vi "Control Panel.vi"(8 "error in (no error)":errorcluster, 11 "Fake Fluke Multimeter in":refnum<class "Fluke Multimeter.lvclass">) -> (0 "error out":errorcluster, 3 "Fake Fluke Multimeter out":refnum<class "Fluke Multimeter.lvclass">)   [LabVIEW 2017, in "Fluke Multimeter.lvclass"]
doc: "(Dynamic) A user-level application that simulates the physical front panel of the Instrument. Provide the user with buttons to manually control features of the instrument, and provide indicators of its current state."
uses:
  Fluke Multimeter.lvclass
  Fluke Multimeter.lvclass/Fluke Multimeter.ctl
  Fluke 8840/Fluke 8840.lvlib
  Utility Classes/Readable/Readable.lvclass
panel:
  out "AutoRange":bool
  out "unit":string
  in  "Reset":bool
  in  "Read Current Value":bool
  out "Value":dbl
  in  "Set":bool
  in  "Read to Control":bool
  in  "Read":bool
  in  "trigger mode set":u16(ring) items=["internal - continuous trigger", "external - rear panel trigger with delay", "external - bus trigger with delay", "external - rear panel trigger", "external - bus trigger"]
  in  "rate set":u16(ring) items=["slow", "medium", "fast"]
  in  "range set":u16(ring)=6 items=["autorange", "200mV, 200 ohms", "2V, 2 kohms", "20V, 20 kohms", "200V, 200 kohms", "1000Vdc, 700 Vac, 2 Mohms", "20 Mohms"]
  in  "function set":u16(ring) items=["volts DC", "volts AC", "2-wire k.ohms", "4-wire k.ohms", "mA DC", "mA AC"]
  out "trigger mode":u16(ring) items=["internal - continuous trigger", "external - rear panel trigger with delay", "external - bus trigger with delay", "external - rear panel trigger", "external - bus trigger"]
  out "rate":u16(ring) items=["slow", "medium", "fast"]
  out "range":u16(ring)=6 items=["autorange", "200mV, 200 ohms", "2V, 2 kohms", "20V, 20 kohms", "200V, 200 kohms", "1000Vdc, 700 Vac, 2 Mohms", "20 Mohms"]
  out "function":u16(ring) items=["volts DC", "volts AC", "2-wire k.ohms", "4-wire k.ohms", "mA DC", "mA AC"]
  in  "stop":bool
  in  "Copy actual to set":bool
  in  "Populate fields with member data":bool
  # "Note: can't set trigger mode yet. Apparently need to create driver for the Y1 command"
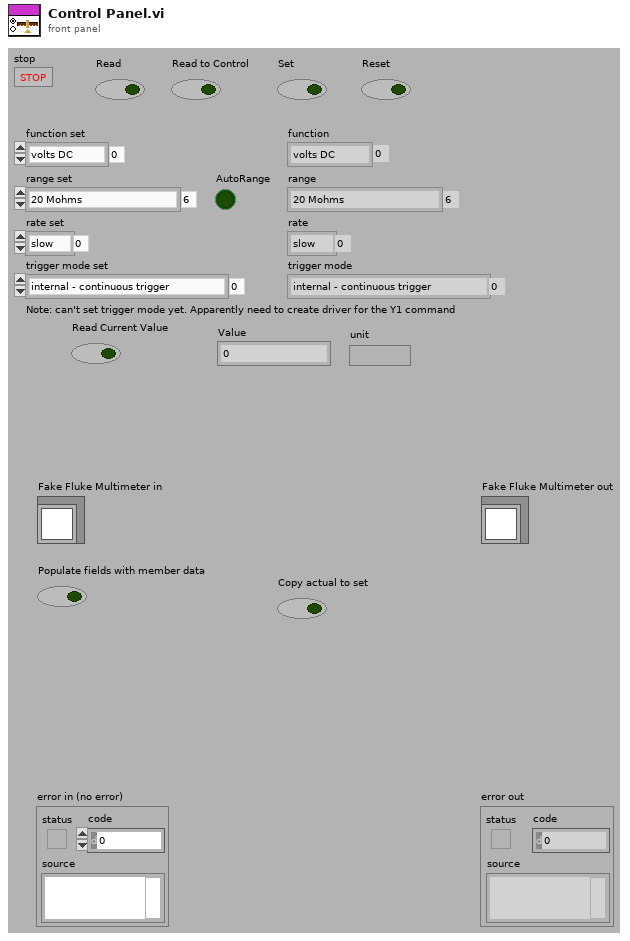
[diagram p1: front panel]
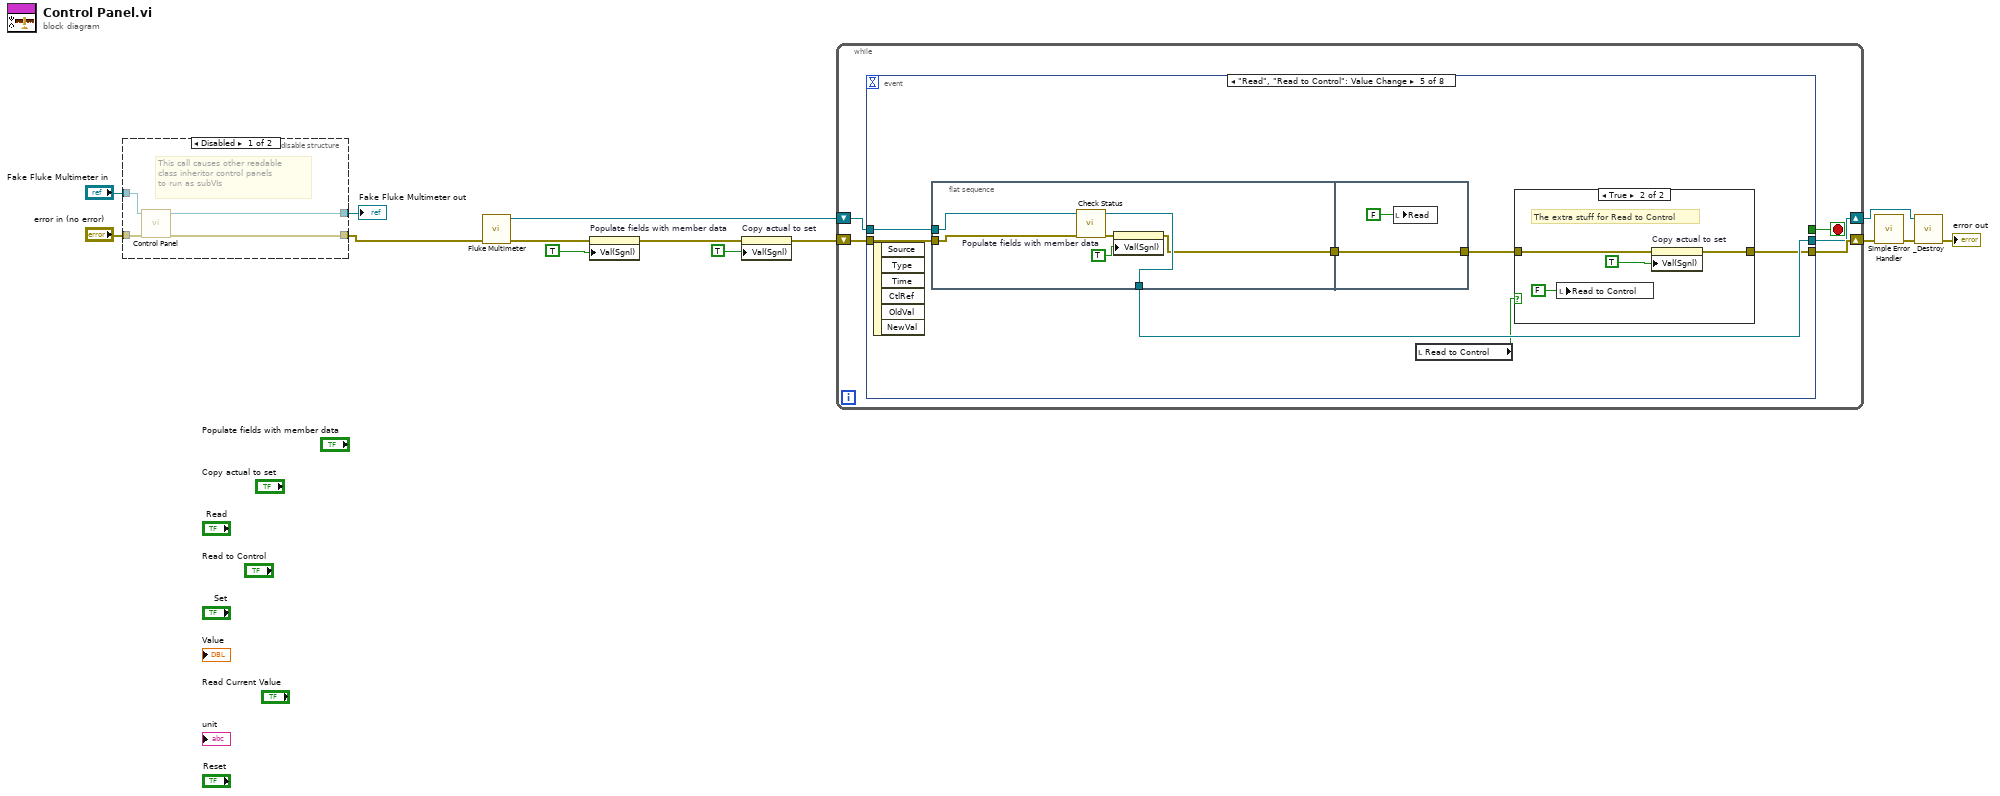
[diagram p0: block diagram]
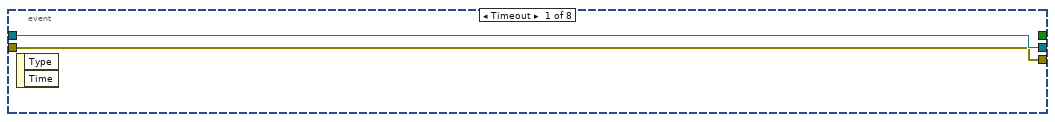
[diagram p3: hidden frame]
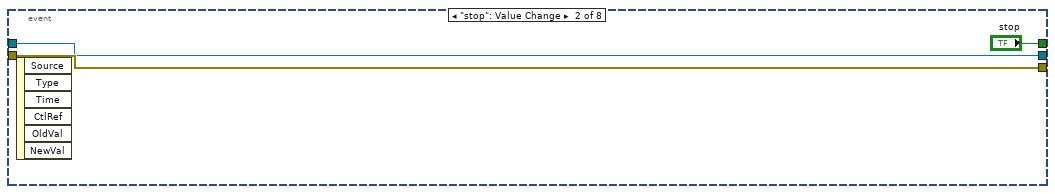
[diagram p4: hidden frame]
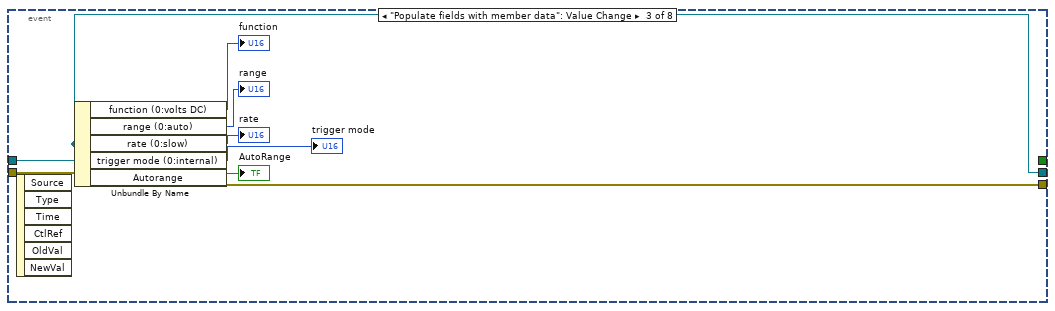
[diagram p5: hidden frame]
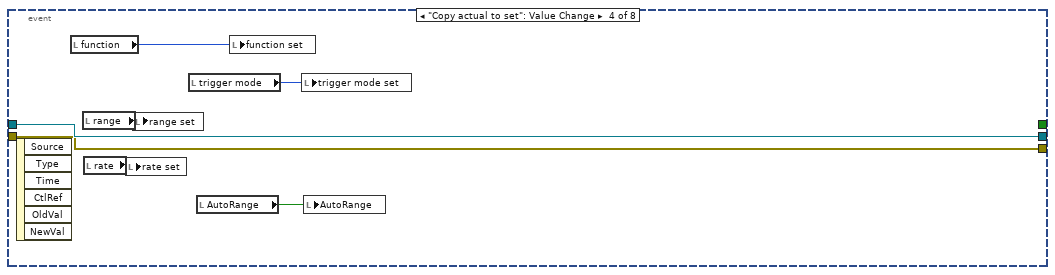
[diagram p6: hidden frame]
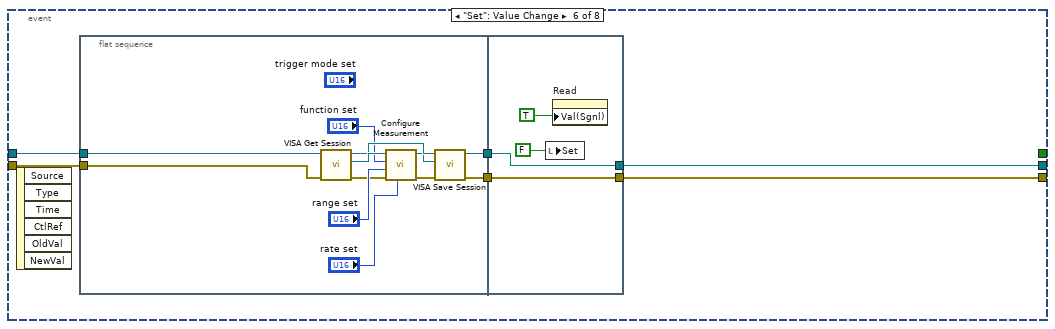
[diagram p8: hidden frame]
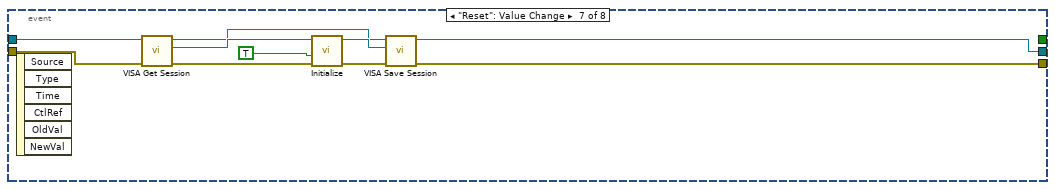
[diagram p9: hidden frame]
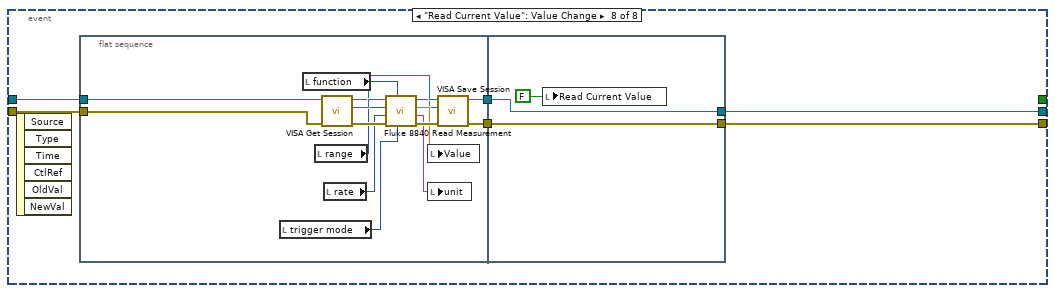
[diagram p10: hidden frame]
diagram:
  n1 = disable-structure shown="Disabled" {
    disable-tunnel: [w18 w20] -> w14
    disable-tunnel: "error in (no error)" -> [w17 w19]
    disable-tunnel: "Fake Fluke Multimeter in" -> [w16 w20]
    disable-tunnel: [w15 w19] -> w11
    frame Disabled {
      # "This call causes other readable\nclass inheritor control panels\nto run as subVIs"
      n2 = call-parent "Control Panel.vi"("error in (no error)"=w17, "Instrument in"=w16) -> ("error out"=w15:errorcluster, "Instrument out"=w18:refnum<class "Fluke Multimeter.lvclass">)  [unwired: 8 out]
    }
    frame Enabled {
    }
  }
  "Fake Fluke Multimeter out" <- w14
  n3 = call "Fluke Multimeter.vi"("error in (no error)"=w11) -> ("error out"=w10:errorcluster, "Fluke Multimeter out"=w7:refnum<class "Fluke Multimeter.lvclass">)  [unwired: 9 out]
  n4 = property on="Populate fields with member data" class="Bool (strict)"(error in=w10, "Val(Sgnl)"=TRUE ("Value (Signaling)")) -> (error out=w9:errorcluster)  [unwired: 1 in, 1 out]
  n5 = property on="Copy actual to set" class="Bool (strict)"(error in=w9, "Val(Sgnl)"=TRUE ("Value (Signaling)")) -> (error out=w8:errorcluster)  [unwired: 1 in, 1 out]
  n6 = while {
    shift-right: [w22] -> w5
    shift-left: w7 -> [w21]
    shift-right: [w24] -> w2
    shift-left: w8 -> [w23]
    stop <- w25 stop-if-true
    n7 = event shown="[4] \"Read\", \"Read to Control\": Value Change" {
      selector: _ -> [_ _ _ _ _ _ _ _]
      dyn-events: _ -> [_ _ _ _ _ _ _ _]
      timeout: _ -> [_ _ _ _ _ _ _ _]
      tunnel: [_ "stop" _ _ _ _ _ _] -> w25
      tunnel: [w26 w29 w32 w39 w45 w67 w88 w100] -> w24
      tunnel: w23 -> [w26 w29 w32 w39 w51 w69 w93 w99]
      tunnel: [w27 w28 w33 w40 w49 w68 w87 w101] -> w22
      tunnel: w21 -> [w27 w28 w33 w40 w50 w70 w94 w102]
      event Timeout {
        n8 = event-data() -> ()  [unwired: 3 out]
      }
      event "stop": Value Change {
        n9 = event-data() -> ()  [unwired: 7 out]
      }
      event "Populate fields with member data": Value Change {
        n10 = event-data() -> ()  [unwired: 7 out]
        n11 = Unbundle By Name(w33) -> ("function (0:volts DC)"=→"function":u16, "range (0:auto)"=→"range":u16, "rate (0:slow)"=→"rate":u16, "trigger mode (0:internal)"=→"trigger mode":u16, "Autorange"=→"AutoRange":bool)
      }
      event "Copy actual to set": Value Change {
        n12 = event-data() -> ()  [unwired: 7 out]
        n13 = local read "function"() -> (w44:u16)
        n14 = local read "range"() -> (w43:u16)
        n15 = local read "rate"() -> (w42:u16)
        n16 = local write "rate set"(w42) -> ()
        n17 = local write "range set"(w43) -> ()
        n18 = local read "trigger mode"() -> (w41:u16)
        n19 = local read "AutoRange"() -> (w38:bool)
        n20 = local write "function set"(w44) -> ()
        n21 = local write "trigger mode set"(w41) -> ()
        n22 = local write "AutoRange"(w38) -> ()
      }
      event "Read", "Read to Control": Value Change {
        n23 = event-data() -> ()  [unwired: 7 out]
        n24 = flat-sequence {
          tunnel: w51 -> [w62]
          tunnel: w50 -> [w61]
          tunnel: [w60] -> w49
          tunnel: [w57] -> w46
          tunnel: [w63] -> w47
          tunnel: w46 -> [w63]
          frame #0 {
            n25 = call-dynamic "Check Status.vi"("error in (no error)"=w62, "Fluke Multimeter in"=w61) -> ("error out"=w59:errorcluster, "Fluke Multimeter out"=w60:refnum<class "Fluke Multimeter.lvclass">)  [unwired: 8 out]
            n26 = property on="Populate fields with member data" class="Bool (strict)"(error in=w59, "Val(Sgnl)"=TRUE ("Value (Signaling)")) -> (error out=w57:errorcluster)  [unwired: 1 in, 1 out]
          }
          frame #1 {
            n27 = local write "Read"(FALSE ("Read")) -> ()
          }
        }
        n28 = local read "Read to Control"() -> (w48:bool)
        n29 = case shown="True" w48 {
          tunnel: w47 -> [w52 w54]
          tunnel: [w52 w53] -> w45
          frame False {
          }
          frame True {
            # "The extra stuff for Read to Control"
            n30 = local write "Read to Control"(FALSE ("Read to Control")) -> ()
            n31 = property on="Copy actual to set" class="Bool (strict)"(error in=w54, "Val(Sgnl)"=TRUE ("Value (Signaling)")) -> (error out=w53:errorcluster)  [unwired: 1 in, 1 out]
          }
        }
      }
      event "Set": Value Change {
        n32 = event-data() -> ()  [unwired: 7 out]
        n33 = flat-sequence {
          tunnel: w70 -> [w82]
          tunnel: w69 -> [w81]
          tunnel: [w78] -> w66
          tunnel: [w71] -> w65
          tunnel: [w85] -> w67
          tunnel: [w86] -> w68
          tunnel: w66 -> [w86]
          tunnel: w65 -> [w85]
          frame #0 {
            n34 = call-dynamic "VISA Get Session.vi"("error in (no error)"=w81, "Instrument.lvclass in"=w82) -> ("error out"=w75:errorcluster, "VISA Resource Name"=w80:refnum<visa-resource-name>, "Instrument.lvclass out"=w79:refnum<class "Fluke Multimeter.lvclass">)  [unwired: 7 out]
            n35 = call "Configure Measurement.vi"("rate (0:slow)"="rate set", "error in (no error)"=w75, "range (0:auto)"="range set", "function (0:volts DC)"="function set", "VISA resource name"=w80) -> ("error out"=w74:errorcluster, "VISA resource name out"=w73:refnum<visa-resource-name>)  [unwired: 5 out]
            n36 = call-dynamic "VISA Save Session.vi"("error in (no error)"=w74, "VISA Resource Name"=w73, "Instrument.lvclass in"=w79) -> ("error out"=w71:errorcluster, "Instrument.lvclass out"=w78:refnum<class "Fluke Multimeter.lvclass">)  [unwired: 7 out]
          }
          frame #1 {
            n37 = local write "Set"(FALSE ("Set")) -> ()
            n38 = property on="Read" class="Bool (strict)"("Val(Sgnl)"=TRUE ("Value (Signaling)")) -> ()  [unwired: 2 in, 2 out]
          }
        }
      }
      event "Reset": Value Change {
        n39 = event-data() -> ()  [unwired: 7 out]
        n40 = call-dynamic "VISA Get Session.vi"("error in (no error)"=w93, "Instrument.lvclass in"=w94) -> ("error out"=w90:errorcluster, "VISA Resource Name"=w92:refnum<visa-resource-name>, "Instrument.lvclass out"=w91:refnum<class "Fluke Multimeter.lvclass">)  [unwired: 7 out]
        n41 = call "Initialize.vi"("error in (no error)"=w90, "reset (T:yes)"=TRUE, "VISA resource name"=w92) -> ("error out"=w89:errorcluster, "VISA resource name out"=w95:refnum<visa-resource-name>)  [unwired: 7 out]
        n42 = call-dynamic "VISA Save Session.vi"("error in (no error)"=w89, "VISA Resource Name"=w95, "Instrument.lvclass in"=w91) -> ("error out"=w88:errorcluster, "Instrument.lvclass out"=w87:refnum<class "Fluke Multimeter.lvclass">)  [unwired: 7 out]
      }
      event "Read Current Value": Value Change {
        n43 = event-data() -> ()  [unwired: 7 out]
        n44 = flat-sequence {
          tunnel: w102 -> [w116]
          tunnel: w99 -> [w103]
          tunnel: [w114] -> w98
          tunnel: [w105] -> w97
          tunnel: [w119] -> w100
          tunnel: [w120] -> w101
          tunnel: w98 -> [w120]
          tunnel: w97 -> [w119]
          frame #0 {
            n45 = local read "trigger mode"() -> (w111:u16)
            n46 = local read "function"() -> (w108:u16)
            n47 = local read "range"() -> (w109:u16)
            n48 = call-dynamic "VISA Get Session.vi"("error in (no error)"=w103, "Instrument.lvclass in"=w116) -> ("error out"=w113:errorcluster, "VISA Resource Name"=w117:refnum<visa-resource-name>, "Instrument.lvclass out"=w115:refnum<class "Fluke Multimeter.lvclass">)  [unwired: 7 out]
            n49 = local read "rate"() -> (w110:u16)
            n50 = call "Fluke 8840 Read Measurement.vi"("trigger mode (0:internal)"=w111, "function (0:volts DC)"=w108, "error in (no error)"=w113, "rate (0:slow)"=w110, "range (0:auto)"=w109, "VISA resource name"=w117) -> ("error out"=w112:errorcluster, "unit"=w104:string, "measurement"=w107:dbl, "VISA resource name out"=w106:refnum<visa-resource-name>)  [unwired: 2 out]
            n51 = local write "Value"(w107) -> ()
            n52 = local write "unit"(w104) -> ()
            n53 = call-dynamic "VISA Save Session.vi"("error in (no error)"=w112, "VISA Resource Name"=w106, "Instrument.lvclass in"=w115) -> ("error out"=w105:errorcluster, "Instrument.lvclass out"=w114:refnum<class "Fluke Multimeter.lvclass">)  [unwired: 7 out]
          }
          frame #1 {
            n54 = local write "Read Current Value"(FALSE ("Read Current Value")) -> ()
          }
        }
      }
    }
  }
  n55 = call <vilib>:"Simple Error Handler.vi"("error in (no error)"=w2) -> ("error out"=w1:errorcluster)  [unwired: 1 in, 7 out]
  n56 = call-dynamic "_Destroy.vi"("error in (no error)"=w1, "Instrument in"=w5) -> ("error out"=→"error out":errorcluster)  [unwired: 9 out]
